vi "NRZ Encoder.vi"() -> ()   [LabVIEW 2026]
panel:
  out "NRZ Output":dbl
  in  "Input Bit":i32
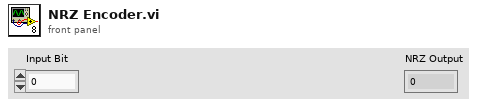
[diagram p1: front panel]
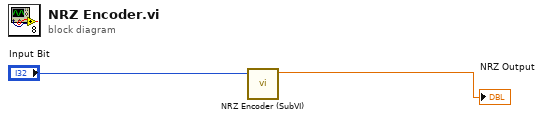
[diagram p0: block diagram]
diagram:
  n1 = call "NRZ Encoder (SubVI).vi"("Input Bit"="Input Bit") -> ("NRZ Output"=→"NRZ Output":dbl)  [unwired: 10 in]
